vi "TestM1M3SALCommands.vi"() -> ()   [LabVIEW 2016]
uses:
  DataTypes/Topics/Parts/CommandId.ctl
  Communicator/M1M3SAL/M1M3SAL.lvclass
  Communicator/DataTypes/M1M3SALSettings.ctl
  UserEvents/UserEvents.lvclass
  DataTypes/General/ShutdownEvent.ctl
  Communicator/M1M3SAL/M1M3SAL.lvclass/M1M3SAL.ctl
  UserEvents/UserEvents.lvclass/UserEvents.ctl
  Commands/AbortLowerM1M3Command/AbortLowerM1M3Command.lvclass
  Commands/AbortLowerM1M3Command/AbortLowerM1M3Command.lvclass/AbortLowerM1M3Command.ctl
  Commands/AbortRaiseM1M3Command/AbortRaiseM1M3Command.lvclass
  Commands/AbortRaiseM1M3Command/AbortRaiseM1M3Command.lvclass/AbortRaiseM1M3Command.ctl
  Commands/ApplyAberrationByBendingModesCommand/ApplyAberrationByBendingModesCommand.lvclass
  Commands/ApplyAberrationByBendingModesCommand/ApplyAberrationByBendingModesCommand.lvclass/ApplyAberrationByBendingModesCommand.ctl
  Commands/ApplyAberrationByForcesCommand/ApplyAberrationByForcesCommand.lvclass
  Commands/ApplyAberrationByForcesCommand/ApplyAberrationByForcesCommand.lvclass/ApplyAberrationByForcesCommand.ctl
  Commands/ApplyAOSCorrectionByBendingModesCommand/ApplyAOSCorrectionByBendingModesCommand.lvclass
  Commands/ApplyAOSCorrectionByBendingModesCommand/ApplyAOSCorrectionByBendingModesCommand.lvclass/ApplyAOSCorrectionByBendingModesCommand.ctl
  Commands/ApplyAOSCorrectionByForcesCommand/ApplyAOSCorrectionByForcesCommand.lvclass
  Commands/ApplyAOSCorrectionByForcesCommand/ApplyAOSCorrectionByForcesCommand.lvclass/ApplyAOSCorrectionByForcesCommand.ctl
  Commands/ClearAberrationCommand/ClearAberrationCommand.lvclass
  Commands/ClearAberrationCommand/ClearAberrationCommand.lvclass/ClearAberrationCommand.ctl
  Commands/ClearAOSCorrectionCommand/ClearAOSCorrectionCommand.lvclass
  Commands/ClearAOSCorrectionCommand/ClearAOSCorrectionCommand.lvclass/ClearAOSCorrectionCommand.ctl
  Commands/DisableCommand/DisableCommand.lvclass
  Commands/DisableCommand/DisableCommand.lvclass/DisableCommand.ctl
  Commands/EnableCommand/EnableCommand.lvclass
  Commands/EnableCommand/EnableCommand.lvclass/EnableCommand.ctl
  Commands/EnterMaintenanceCommand/EnterMaintenanceCommand.lvclass
  Commands/EnterMaintenanceCommand/EnterMaintenanceCommand.lvclass/EnterMaintenanceCommand.ctl
  Commands/ExitCommand/ExitCommand.lvclass
  Commands/ExitCommand/ExitCommand.lvclass/ExitCommand.ctl
  Commands/ExitMaintenanceCommand/ExitMaintenanceCommand.lvclass
  Commands/ExitMaintenanceCommand/ExitMaintenanceCommand.lvclass/ExitMaintenanceCommand.ctl
  Commands/LowerM1M3Command/LowerM1M3Command.lvclass
  Commands/LowerM1M3Command/LowerM1M3Command.lvclass/LowerM1M3Command.ctl
  Commands/ManipulateM1M3Command/ManipulateM1M3Command.lvclass
  Commands/ManipulateM1M3Command/ManipulateM1M3Command.lvclass/ManipulateM1M3Command.ctl
  Commands/MoveHardpointActuatorsCommand/MoveHardpointActuatorsCommand.lvclass
  Commands/MoveHardpointActuatorsCommand/MoveHardpointActuatorsCommand.lvclass/MoveHardpointActuatorsCommand.ctl
  Commands/RaiseM1M3Command/RaiseM1M3Command.lvclass
  Commands/RaiseM1M3Command/RaiseM1M3Command.lvclass/RaiseM1M3Command.ctl
  Commands/ShutdownCommand/ShutdownCommand.lvclass
  Commands/ShutdownCommand/ShutdownCommand.lvclass/ShutdownCommand.ctl
  Commands/StandbyCommand/StandbyCommand.lvclass
  Commands/StandbyCommand/StandbyCommand.lvclass/StandbyCommand.ctl
  Commands/StartCommand/StartCommand.lvclass
  Commands/StartCommand/StartCommand.lvclass/StartCommand.ctl
  Commands/TestAirCommand/TestAirCommand.lvclass
  Commands/TestAirCommand/TestAirCommand.lvclass/TestAirCommand.ctl
  Commands/TestForceActuatorCommand/TestForceActuatorCommand.lvclass
  Commands/TestForceActuatorCommand/TestForceActuatorCommand.lvclass/TestForceActuatorCommand.ctl
  Commands/TestHardpointCommand/TestHardpointCommand.lvclass
  Commands/TestHardpointCommand/TestHardpointCommand.lvclass/TestHardpointCommand.ctl
  DataTypes/Topics/CommandStart.ctl
  DataTypes/Topics/CommandEnable.ctl
  DataTypes/Topics/CommandDisable.ctl
  DataTypes/Topics/CommandStandby.ctl
  DataTypes/Topics/CommandShutdown.ctl
  DataTypes/Topics/CommandExit.ctl
  DataTypes/Topics/CommandManipulateM1M3.ctl
  DataTypes/Topics/CommandTestAir.ctl
  DataTypes/Topics/CommandEnterMaintenance.ctl
  DataTypes/Topics/CommandExitMaintenance.ctl
  DataTypes/Topics/CommandTestHardpoint.ctl
  DataTypes/Topics/CommandTestForceActuator.ctl
  DataTypes/Topics/CommandMoveHardpointActuators.ctl
  DataTypes/Topics/CommandClearAOSCorrection.ctl
  DataTypes/Topics/CommandApplyAOSCorrectionByBendingModes.ctl
  DataTypes/Topics/CommandApplyAOSCorrectionByForces.ctl
  DataTypes/Topics/CommandAbortLowerM1M3.ctl
  DataTypes/Topics/CommandAbortRaiseM1M3.ctl
  DataTypes/Topics/CommandRaiseM1M3.ctl
  DataTypes/Topics/CommandLowerM1M3.ctl
  DataTypes/Topics/CommandApplyAberrationByForces.ctl
  DataTypes/Topics/CommandApplyAberrationByBendingModes.ctl
  DataTypes/Topics/CommandClearAberration.ctl
  Communicator/M1M3SupportCommunicator.lvlib
  DataTypes/General/M1M3SupportGeneral.lvlib
  DataTypes/Topics/M1M3SupportTopics.lvlib
  Commands/Command/Command.lvclass
panel:
  out "CommandId":T1
  out "SAL Start Time (s)":dbl format="%.6g"
  out "ClearAberration":bool
  out "ApplyAberrationBModes":bool
  out "ApplyAberrationForces":bool
  out "Lower":bool
  out "Raise":bool
  out "AbortRaise":bool
  out "AbortLower":bool
  out "ApplyAOSForces":bool
  out "ApplyAOSBModes":bool
  out "ClearAOSCorrection":bool
  out "MoveHardpointActuators":bool
  out "TestForceActuator":bool
  out "TestHardpoint":bool
  in  "ClearAberrationGo":bool
  in  "ApplyAberrationBModesGo":bool
  in  "ApplyAberrationForcesGo":bool
  in  "LowerGo":bool
  in  "RaiseGo":bool
  in  "AbortRaiseGo":bool
  in  "AbortLowerGo":bool
  in  "ApplyAOSForcesGo":bool
  in  "ApplyAOSBModesGo":bool
  in  "ClearAOSCorrectionGo":bool
  in  "MoveHardpointActuatorsGo":bool
  in  "TestForceActuatorGo":bool
  in  "TestHardpointGo":bool
  out "TestAir":bool
  in  "TestAirGo":bool
  out "ExitMaintenance":bool
  out "EnterMaintenance":bool
  out "ManipulateM1M3":bool
  in  "ExitMaintenanceGo":bool
  in  "EnterMaintenanceGo":bool
  in  "ManipulateM1M3Go":bool
  out "Exit":bool
  out "Shutdown":bool
  out "Standby":bool
  out "Disable":bool
  in  "ExitGo":bool
  in  "ShutdownGo":bool
  in  "StandbyGo":bool
  in  "DisableGo":bool
  in  "EnableGo":bool
  out "Enable":bool
  out "Ready?":bool
  in  "StartGo":bool
  out "Start":bool
  in  "Stop":bool
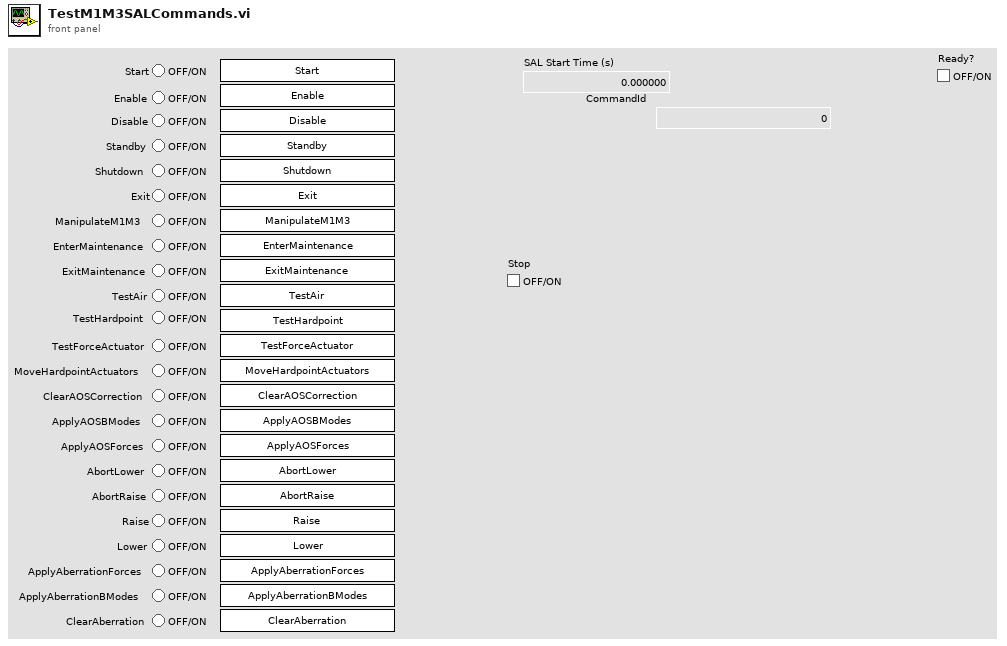
[diagram p1: front panel]
types:
  T1 = typedef "M1M3SupportTopics.lvlib/CommandId.ctl" = i32
  T2 = typedef "M1M3SupportGeneral.lvlib/ShutdownEvent.ctl" = cluster{"Shutdown":bool}
  T3 = typedef "M1M3SupportCommunicator.lvlib/M1M3SALSettings.ctl" = cluster{"IPAddress":string, "Port":u16, "StartupScript":string}
  T4 = typedef "M1M3SupportTopics.lvlib/CommandAbortLowerM1M3.ctl" = cluster{"CommandId":T1, "AbortLowerM1M3":bool}
  T5 = typedef "M1M3SupportTopics.lvlib/CommandAbortRaiseM1M3.ctl" = cluster{"CommandId":T1, "AbortRaiseM1M3":bool}
  T6 = typedef "M1M3SupportTopics.lvlib/CommandApplyAberrationByBendingModes.ctl" = cluster{"CommandId":T1, "Coefficients":dbl[]}
  T7 = typedef "M1M3SupportTopics.lvlib/CommandApplyAberrationByForces.ctl" = cluster{"CommandId":T1, "ZForces":dbl[]}
  T8 = typedef "M1M3SupportTopics.lvlib/CommandApplyAOSCorrectionByBendingModes.ctl" = cluster{"CommandId":T1, "Coefficients":dbl[]}
  T9 = typedef "M1M3SupportTopics.lvlib/CommandApplyAOSCorrectionByForces.ctl" = cluster{"CommandId":T1, "ZForces":dbl[]}
  T10 = typedef "M1M3SupportTopics.lvlib/CommandClearAberration.ctl" = cluster{"CommandId":T1, "ClearAberration":bool}
  T11 = typedef "M1M3SupportTopics.lvlib/CommandClearAOSCorrection.ctl" = cluster{"CommandId":T1, "ClearAOSCorrection":bool}
  T12 = typedef "M1M3SupportTopics.lvlib/CommandDisable.ctl" = cluster{"CommandId":T1, "Disable":bool}
  T13 = typedef "M1M3SupportTopics.lvlib/CommandEnable.ctl" = cluster{"CommandId":T1, "Enable":bool}
  T14 = typedef "M1M3SupportTopics.lvlib/CommandEnterMaintenance.ctl" = cluster{"CommandId":T1, "EnterMaintenance":bool}
  T15 = typedef "M1M3SupportTopics.lvlib/CommandExit.ctl" = cluster{"CommandId":T1, "Exit":bool}
  T16 = typedef "M1M3SupportTopics.lvlib/CommandExitMaintenance.ctl" = cluster{"CommandId":T1, "ExitMaintenance":bool}
  T17 = typedef "M1M3SupportTopics.lvlib/CommandLowerM1M3.ctl" = cluster{"CommandId":T1, "LowerM1M3":bool}
  T18 = typedef "M1M3SupportTopics.lvlib/CommandManipulateM1M3.ctl" = cluster{"CommandId":T1, "XTranslation":dbl, "YTranslation":dbl, "ZTranslation":dbl, "XRotation":dbl, "YRotation":dbl, "ZRotation":dbl}
  T19 = typedef "M1M3SupportTopics.lvlib/CommandMoveHardpointActuators.ctl" = cluster{"CommandId":T1, "Steps":i8[]}
  T20 = typedef "M1M3SupportTopics.lvlib/CommandRaiseM1M3.ctl" = cluster{"CommandId":T1, "RaiseM1M3":bool}
  T21 = typedef "M1M3SupportTopics.lvlib/CommandShutdown.ctl" = cluster{"CommandId":T1, "Shutdown":bool}
  T22 = typedef "M1M3SupportTopics.lvlib/CommandStandby.ctl" = cluster{"CommandId":T1, "Standby":bool}
  T23 = typedef "M1M3SupportTopics.lvlib/CommandStart.ctl" = cluster{"CommandId":T1, "Start":bool, "SettingToApply":string}
  T24 = typedef "M1M3SupportTopics.lvlib/CommandTestAir.ctl" = cluster{"CommandId":T1, "TestAir":bool}
  T25 = typedef "M1M3SupportTopics.lvlib/CommandTestForceActuator.ctl" = cluster{"CommandId":T1, "ActuatorId":i32}
  T26 = typedef "M1M3SupportTopics.lvlib/CommandTestHardpoint.ctl" = cluster{"CommandId":T1, "ActuatorId":i32}
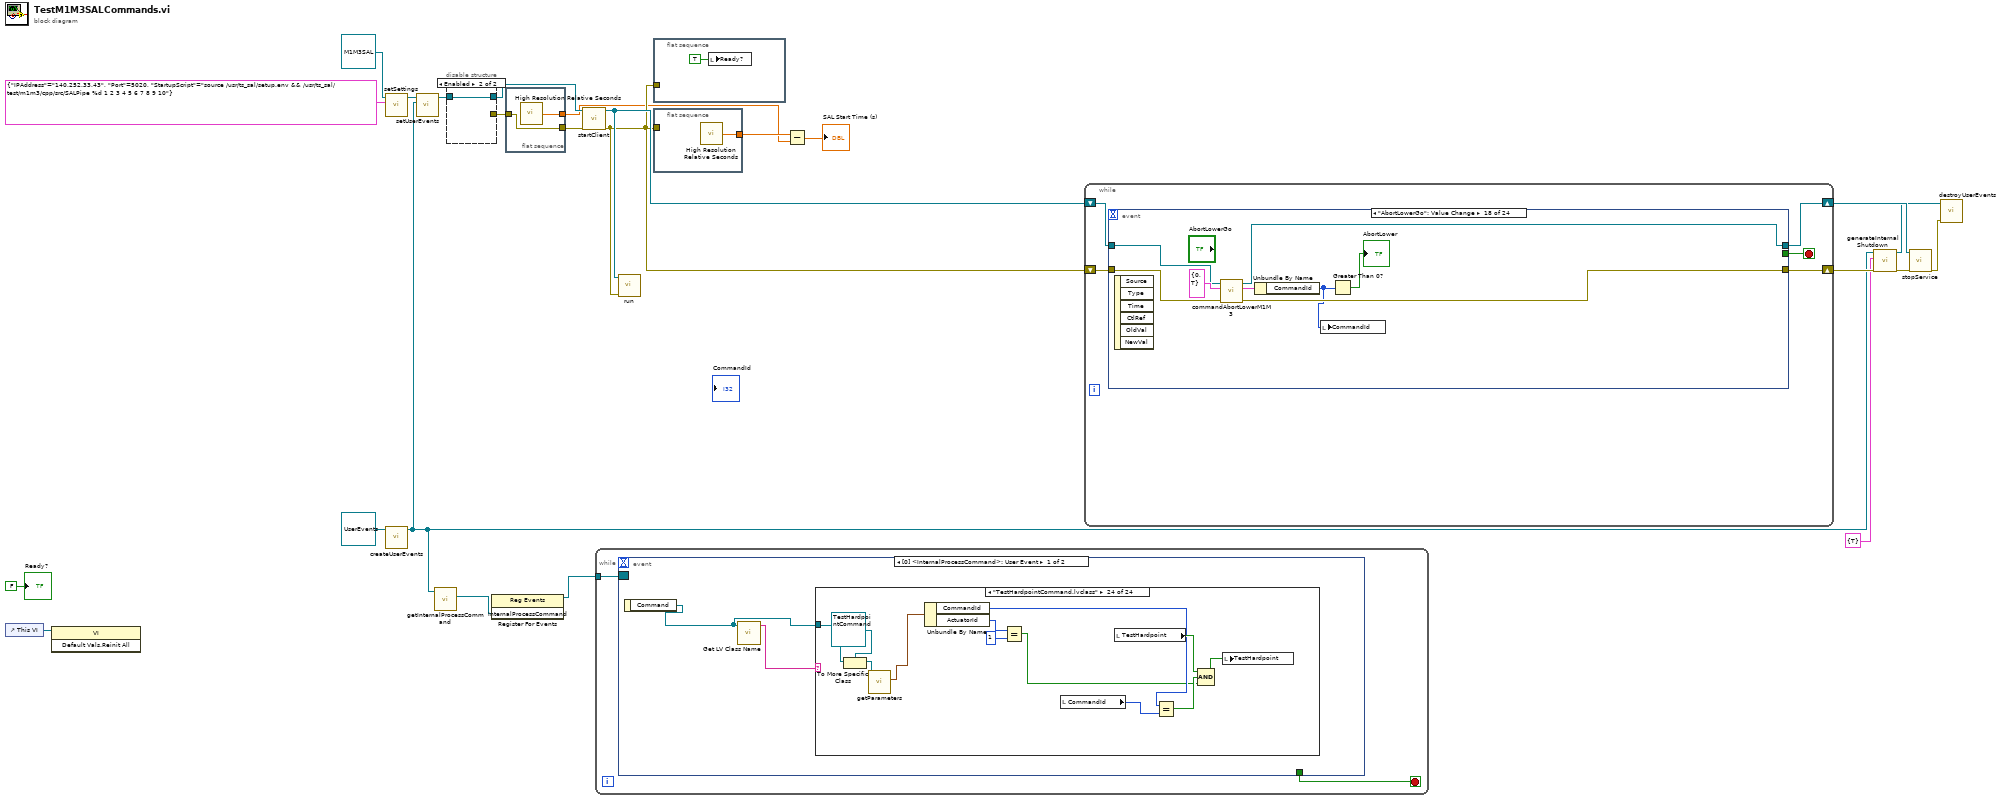
[diagram p0: block diagram]
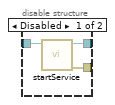
[diagram p2: hidden frame]
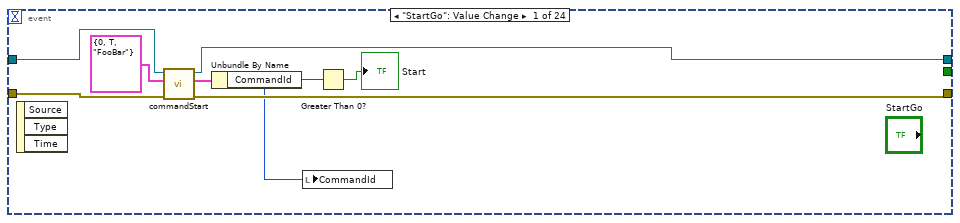
[diagram p3: hidden frame]
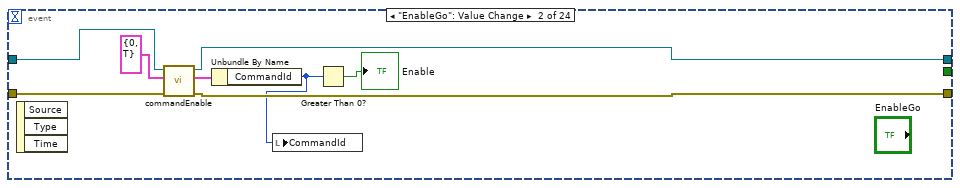
[diagram p4: hidden frame]
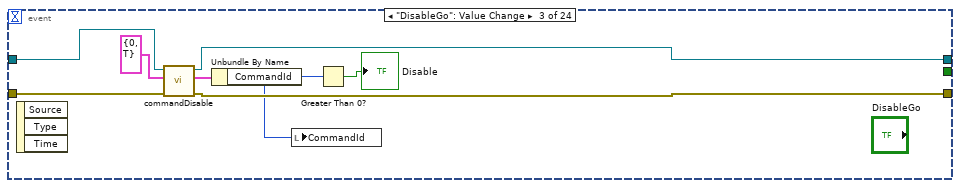
[diagram p5: hidden frame]
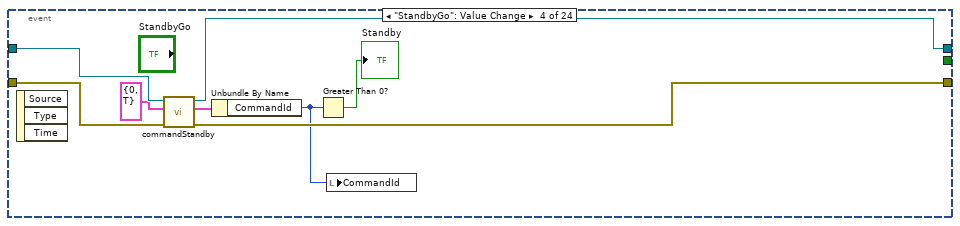
[diagram p6: hidden frame]
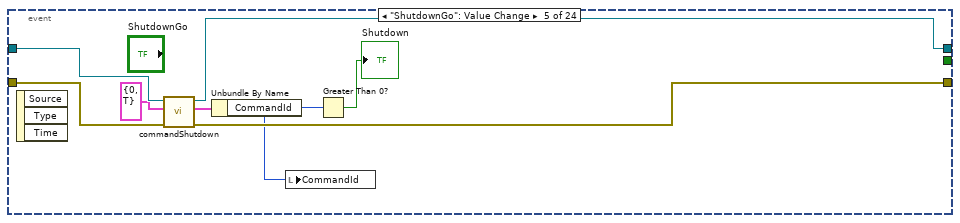
[diagram p7: hidden frame]
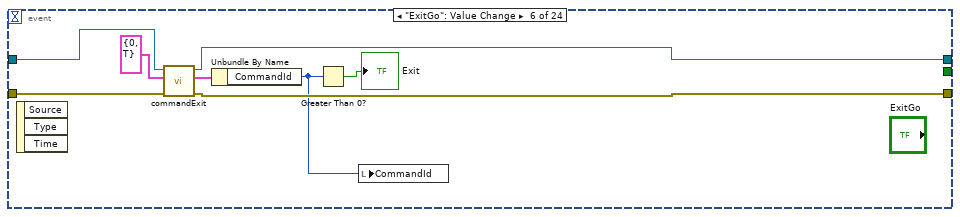
[diagram p8: hidden frame]
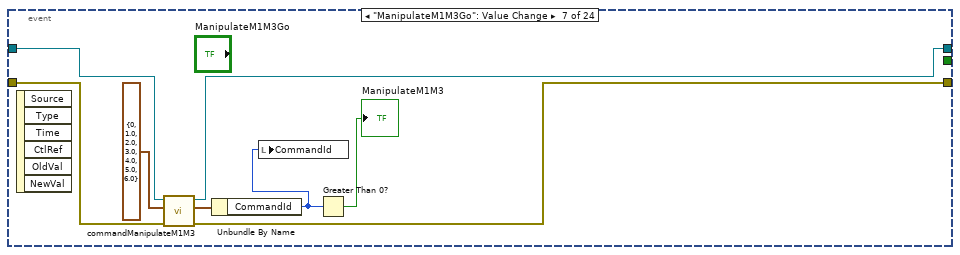
[diagram p9: hidden frame]
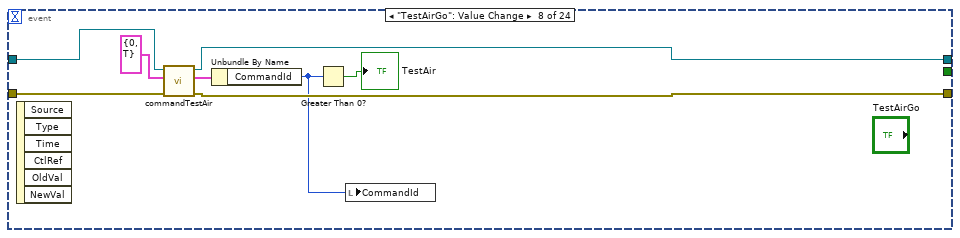
[diagram p10: hidden frame]
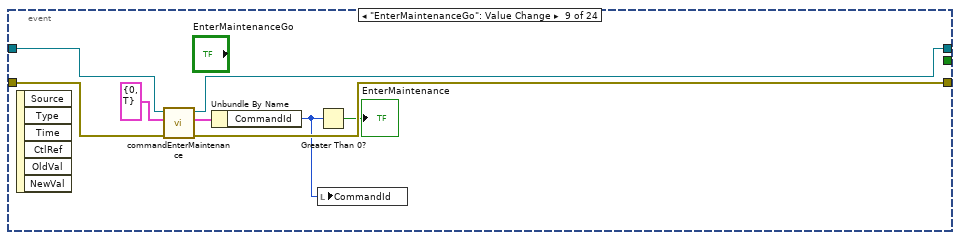
[diagram p11: hidden frame]
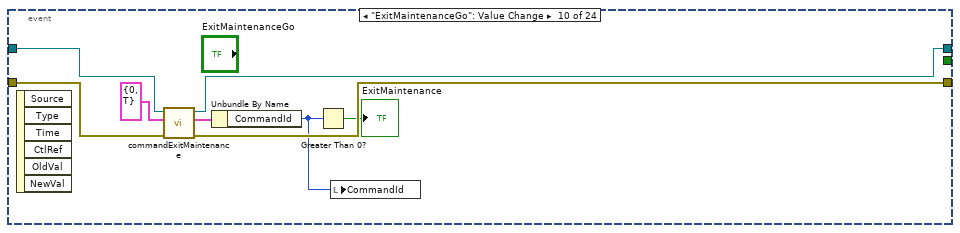
[diagram p12: hidden frame]
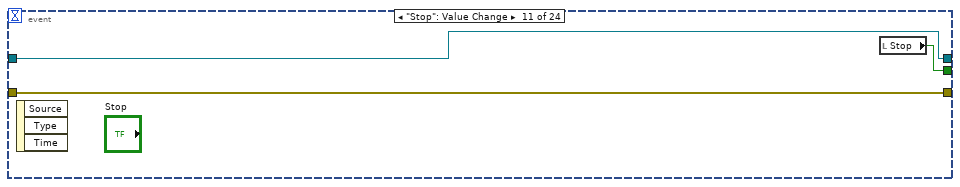
[diagram p13: hidden frame]
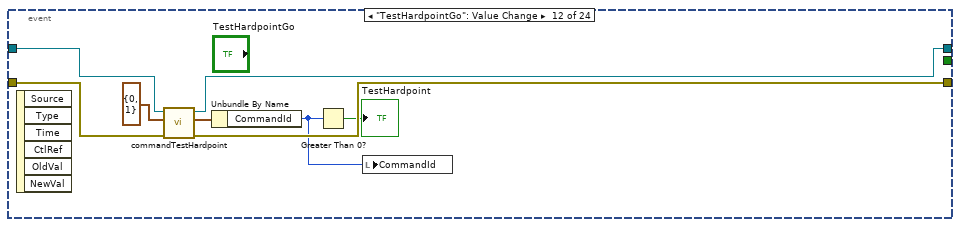
[diagram p14: hidden frame]
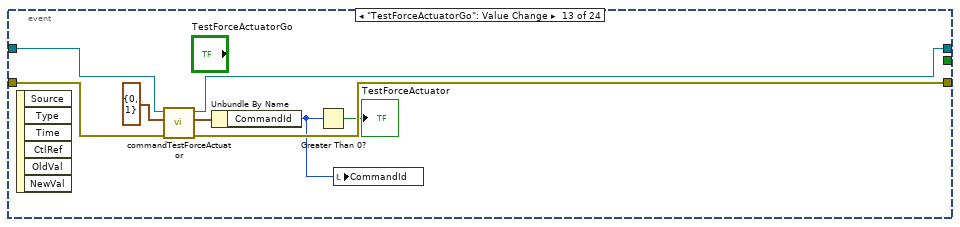
[diagram p15: hidden frame]
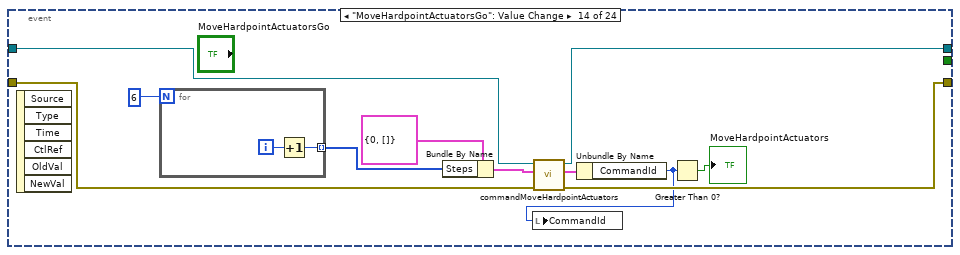
[diagram p16: hidden frame]
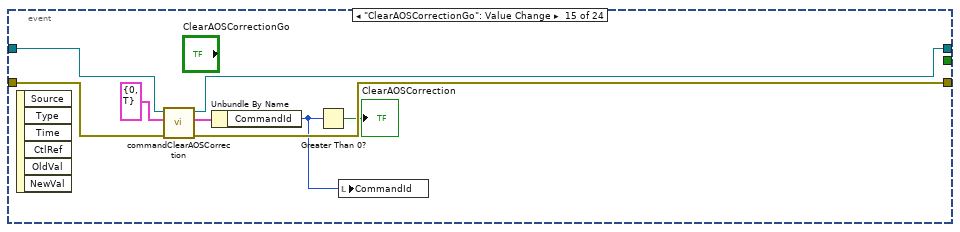
[diagram p17: hidden frame]
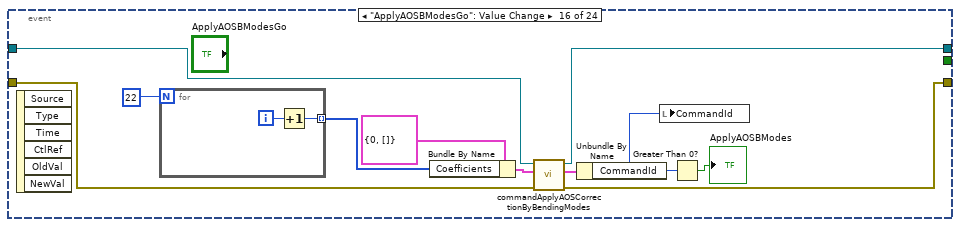
[diagram p18: hidden frame]
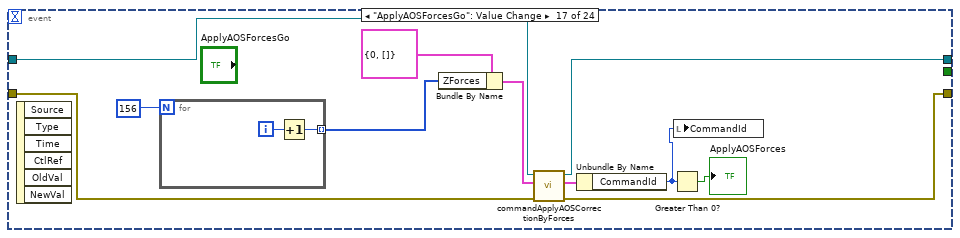
[diagram p19: hidden frame]
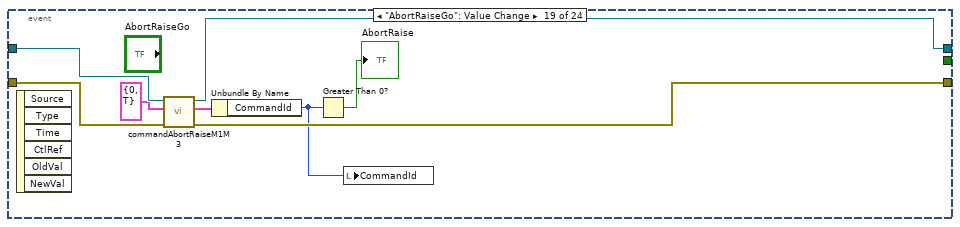
[diagram p20: hidden frame]
diagram:
  n1 = control-ref of="This VI"() -> (w10:refnum<vi>)
  n2 = invoke class="VI" method="Default Vals.Reinit All"(reference=w10) -> ()  [unwired: 2 in, 3 out]
  n3 = call "setSettings.vi"("Settings"=T3 {"IPAddress"="140.252.33.43", "Port"=5020, "StartupScript"="source /usr/ts_sal/setup.env && /usr/ts_sal/test/m1m3/cpp/src/SALPipe %d 1 2 3 4 5 6 7 8 9 10"}, "M1M3SAL in"=refnum<class "M1M3SAL.lvclass"> refnum ("M1M3SupportCommunicator.lvlib:M1M3SAL.lvclass")) -> ("M1M3SAL out"=w21:refnum<class "M1M3SAL.lvclass">)  [unwired: 9 in]
  n4 = call "createUserEvents.vi"("UserEvents in"=refnum<class "UserEvents.lvclass"> refnum ("UserEvents.lvclass")) -> ("UserEvents out"=w3:refnum<class "UserEvents.lvclass">)  [unwired: 9 in, 1 out]
  n5 = call "setUserEvents.vi"("UserEvents"=w3, "M1M3SAL in"=w21) -> ("M1M3SAL out"=w20:refnum<class "M1M3SAL.lvclass">)  [unwired: 9 in]
  n6 = call "getInternalProcessCommand.vi"("UserEvents in"=w3) -> ("InternalProcessCommand"=w2:refnum<user-event>)  [unwired: 9 in, 1 out]
  n7 = disable-structure shown="Enabled" {
    disable-tunnel: w20 -> [w27 w28]
    disable-tunnel: [w26 w28] -> w19
    disable-tunnel: [w25 _] -> w8
    frame Disabled {
      n8 = call-dynamic "startService.vi"("M1M3SAL in"=w27) -> ("error out"=w25:errorcluster, "M1M3SAL out"=w26:refnum<class "M1M3SAL.lvclass">)  [unwired: 9 in]
    }
    frame Enabled {
    }
  }
  n9 = register-events(w2) -> (reference out=w1:refnum<event-registration>)  [unwired: 2 in, 1 out]
  n10 = flat-sequence {
    tunnel: [w30] -> w9
    tunnel: w8 -> [w30]
    tunnel: [w29] -> w5
    frame #0 {
      n11 = call <vilib>:"High Resolution Relative Seconds.vi"() -> ("relative seconds"=w29:dbl)
    }
  }
  n12 = call-dynamic "startClient.vi"("error in (no error)"=w9, "M1M3SAL in"=w19) -> ("error out"=w7:errorcluster, "M1M3SAL out"=w16:refnum<class "M1M3SAL.lvclass">)  [unwired: 8 in]
  n13 = while {
    tunnel: w1 -> [w32]
    stop <- w31 stop-if-true
    n14 = event shown="[0] <InternalProcessCommand>: User Event" {
      selector: w32 -> [_ _]
      dyn-events: _ -> [_ _]
      timeout: _ -> [_ _]
      tunnel: [_ TRUE] -> w31
      event User Event {
        n15 = event-data() -> ("Command"=w33:refnum<class "Command.lvclass">)  [unwired: 1 in]
        n16 = call <vilib>:"Get LV Class Name.vi"("object"=w33) -> ("class name"=w34:string)  [unwired: 9 in, 1 out]
        n17 = case shown="\"TestHardpointCommand.lvclass\"" w34 {
          tunnel: w33 -> [_ w44 w54 w68 w84 w100 w116 w128 w138 w148 w158 w168 w178 w188 w198 w225 w239 w251 w261 w271 w281 w291 w303 w315]
          frame "", Default {
          }
          frame "AbortLowerM1M3Command.lvclass" {
            n18 = To More Specific Class(target class=refnum<class "AbortLowerM1M3Command.lvclass"> refnum ("AbortLowerM1M3Command.lvclass"), reference=w44) -> (specific class reference=w42:refnum<class "AbortLowerM1M3Command.lvclass">)  [unwired: 1 in, 1 out]
            n19 = call "getParameters.vi"("AbortLowerM1M3Command in"=w42) -> ("Parameters"=w41:T4)  [unwired: 9 in, 1 out]
            n20 = local read "CommandId"() -> (w37:T1)
            n21 = Unbundle By Name(w41) -> ("CommandId"=w38:T1, "AbortLowerM1M3"=w40:bool)
            n22 = local read "AbortLower"() -> (w39:bool)
            n23 = Equal?(x=w38, y=w37) -> (x = y?=w36:bool)
            n24 = Compound Arithmetic op=AND(w39, w36, w40) -> (w35:bool)
            n25 = local write "AbortLower"(w35) -> ()
          }
          frame "AbortRaiseM1M3Command.lvclass" {
            n26 = To More Specific Class(target class=refnum<class "AbortRaiseM1M3Command.lvclass"> refnum ("AbortRaiseM1M3Command.lvclass"), reference=w54) -> (specific class reference=w48:refnum<class "AbortRaiseM1M3Command.lvclass">)  [unwired: 1 in, 1 out]
            n27 = call "getParameters.vi"("AbortRaiseM1M3Command in"=w48) -> ("Parameters"=w47:T5)  [unwired: 9 in, 1 out]
            n28 = local read "CommandId"() -> (w52:T1)
            n29 = Unbundle By Name(w47) -> ("CommandId"=w45:T1, "AbortRaiseM1M3"=w46:bool)
            n30 = local read "AbortRaise"() -> (w53:bool)
            n31 = Equal?(x=w45, y=w52) -> (x = y?=w51:bool)
            n32 = Compound Arithmetic op=AND(w53, w51, w46) -> (w50:bool)
            n33 = local write "AbortRaise"(w50) -> ()
          }
          frame "ApplyAberrationByBendingModesCommand.lvclass" {
            n34 = To More Specific Class(target class=refnum<class "ApplyAberrationByBendingModesCommand.lvclass"> refnum ("ApplyAberrationByBendingModesCommand.lvclass"), reference=w68) -> (specific class reference=w61:refnum<class "ApplyAberrationByBendingModesCommand.lvclass">)  [unwired: 1 in, 1 out]
            n35 = for {
              N: 22 -> [_]
              tunnel: [w69] -> w57 mode=indexing
              i -> [w70]
              n36 = Increment(x=w70) -> (x+1=w69:i32)
            }
            n37 = call "getParameters.vi"("ApplyAberrationByBendingModesCommand in"=w61) -> ("Parameters"=w60:T6)  [unwired: 9 in, 1 out]
            n38 = local read "CommandId"() -> (w66:T1)
            n39 = Unbundle By Name(w60) -> ("CommandId"=w63:T1, "Coefficients"=w58:dbl[])
            n40 = Equal?(x=w58, y=w57) -> (x = y?=w56:bool[])
            n41 = And Array Elements(Boolean array=w56) -> (logical AND=w55:bool)
            n42 = local read "ApplyAberrationBModes"() -> (w67:bool)
            n43 = Equal?(x=w63, y=w66) -> (x = y?=w65:bool)
            n44 = Compound Arithmetic op=AND(w67, w65, w55) -> (w64:bool)
            n45 = local write "ApplyAberrationBModes"(w64) -> ()
          }
          frame "ApplyAberrationByForcesCommand.lvclass" {
            n46 = To More Specific Class(target class=refnum<class "ApplyAberrationByForcesCommand.lvclass"> refnum ("ApplyAberrationByForcesCommand.lvclass"), reference=w84) -> (specific class reference=w72:refnum<class "ApplyAberrationByForcesCommand.lvclass">)  [unwired: 1 in, 1 out]
            n47 = call "getParameters.vi"("ApplyAberrationByForcesCommand in"=w72) -> ("Parameters"=w71:T7)  [unwired: 9 in, 1 out]
            n48 = for {
              N: 156 -> [_]
              tunnel: [w85] -> w76 mode=indexing
              i -> [w86]
              n49 = Increment(x=w86) -> (x+1=w85:i32)
            }
            n50 = local read "CommandId"() -> (w82:T1)
            n51 = Unbundle By Name(w71) -> ("CommandId"=w79:T1, "ZForces"=w77:dbl[])
            n52 = Equal?(x=w77, y=w76) -> (x = y?=w75:bool[])
            n53 = And Array Elements(Boolean array=w75) -> (logical AND=w74:bool)
            n54 = local read "ApplyAberrationForces"() -> (w83:bool)
            n55 = Equal?(x=w79, y=w82) -> (x = y?=w81:bool)
            n56 = Compound Arithmetic op=AND(w83, w81, w74) -> (w80:bool)
            n57 = local write "ApplyAberrationForces"(w80) -> ()
          }
          frame "ApplyAOSCorrectionByBendingModesCommand.lvclass" {
            n58 = To More Specific Class(target class=refnum<class "ApplyAOSCorrectionByBendingModesCommand.lvclass"> refnum ("ApplyAOSCorrectionByBendingModesCommand.lvclass"), reference=w100) -> (specific class reference=w88:refnum<class "ApplyAOSCorrectionByBendingModesCommand.lvclass">)  [unwired: 1 in, 1 out]
            n59 = call "getParameters.vi"("ApplyAOSCorrectionByBendingModesCommand in"=w88) -> ("Parameters"=w87:T8)  [unwired: 9 in, 1 out]
            n60 = for {
              N: 22 -> [_]
              tunnel: [w101] -> w92 mode=indexing
              i -> [w102]
              n61 = Increment(x=w102) -> (x+1=w101:i32)
            }
            n62 = local read "CommandId"() -> (w98:T1)
            n63 = Unbundle By Name(w87) -> ("CommandId"=w95:T1, "Coefficients"=w93:dbl[])
            n64 = Equal?(x=w93, y=w92) -> (x = y?=w91:bool[])
            n65 = And Array Elements(Boolean array=w91) -> (logical AND=w90:bool)
            n66 = local read "ApplyAOSBModes"() -> (w99:bool)
            n67 = Equal?(x=w95, y=w98) -> (x = y?=w97:bool)
            n68 = Compound Arithmetic op=AND(w99, w97, w90) -> (w96:bool)
            n69 = local write "ApplyAOSBModes"(w96) -> ()
          }
          frame "ApplyAOSCorrectionByForcesCommand.lvclass" {
            n70 = To More Specific Class(target class=refnum<class "ApplyAOSCorrectionByForcesCommand.lvclass"> refnum ("ApplyAOSCorrectionByForcesCommand.lvclass"), reference=w116) -> (specific class reference=w104:refnum<class "ApplyAOSCorrectionByForcesCommand.lvclass">)  [unwired: 1 in, 1 out]
            n71 = for {
              N: 156 -> [_]
              tunnel: [w117] -> w108 mode=indexing
              i -> [w118]
              n72 = Increment(x=w118) -> (x+1=w117:i32)
            }
            n73 = call "getParameters.vi"("ApplyAOSCorrectionByForcesCommand in"=w104) -> ("Parameters"=w103:T9)  [unwired: 9 in, 1 out]
            n74 = local read "CommandId"() -> (w114:T1)
            n75 = Unbundle By Name(w103) -> ("CommandId"=w111:T1, "ZForces"=w109:dbl[])
            n76 = Equal?(x=w109, y=w108) -> (x = y?=w107:bool[])
            n77 = And Array Elements(Boolean array=w107) -> (logical AND=w106:bool)
            n78 = local read "ApplyAOSForces"() -> (w115:bool)
            n79 = Equal?(x=w111, y=w114) -> (x = y?=w113:bool)
            n80 = Compound Arithmetic op=AND(w115, w113, w106) -> (w112:bool)
            n81 = local write "ApplyAOSForces"(w112) -> ()
          }
          frame "ClearAberrationCommand.lvclass" {
            n82 = To More Specific Class(target class=refnum<class "ClearAberrationCommand.lvclass"> refnum ("ClearAberrationCommand.lvclass"), reference=w128) -> (specific class reference=w121:refnum<class "ClearAberrationCommand.lvclass">)  [unwired: 1 in, 1 out]
            n83 = call "getParameters.vi"("ClearAberrationCommand in"=w121) -> ("Parameters"=w120:T10)  [unwired: 9 in, 1 out]
            n84 = local read "CommandId"() -> (w126:T1)
            n85 = Unbundle By Name(w120) -> ("CommandId"=w123:T1, "ClearAberration"=w119:bool)
            n86 = local read "ClearAberration"() -> (w127:bool)
            n87 = Equal?(x=w123, y=w126) -> (x = y?=w125:bool)
            n88 = Compound Arithmetic op=AND(w127, w125, w119) -> (w124:bool)
            n89 = local write "ClearAberration"(w124) -> ()
          }
          frame "ClearAOSCorrectionCommand.lvclass" {
            n90 = To More Specific Class(target class=refnum<class "ClearAOSCorrectionCommand.lvclass"> refnum ("ClearAOSCorrectionCommand.lvclass"), reference=w138) -> (specific class reference=w129:refnum<class "ClearAOSCorrectionCommand.lvclass">)  [unwired: 1 in, 1 out]
            n91 = call "getParameters.vi"("ClearAOSCorrectionCommand in"=w129) -> ("Parameters"=w131:T11)  [unwired: 9 in, 1 out]
            n92 = local read "CommandId"() -> (w136:T1)
            n93 = Unbundle By Name(w131) -> ("CommandId"=w133:T1, "ClearAOSCorrection"=w132:bool)
            n94 = local read "ClearAOSCorrection"() -> (w137:bool)
            n95 = Equal?(x=w133, y=w136) -> (x = y?=w135:bool)
            n96 = Compound Arithmetic op=AND(w137, w135, w132) -> (w134:bool)
            n97 = local write "ClearAOSCorrection"(w134) -> ()
          }
          frame "DisableCommand.lvclass" {
            n98 = To More Specific Class(target class=refnum<class "DisableCommand.lvclass"> refnum ("DisableCommand.lvclass"), reference=w148) -> (specific class reference=w140:refnum<class "DisableCommand.lvclass">)  [unwired: 1 in, 1 out]
            n99 = call "getParameters.vi"("DisableCommand in"=w140) -> ("Parameters"=w139:T12)  [unwired: 9 in, 1 out]
            n100 = local read "CommandId"() -> (w146:T1)
            n101 = Unbundle By Name(w139) -> ("CommandId"=w143:T1, "Disable"=w142:bool)
            n102 = local read "Disable"() -> (w147:bool)
            n103 = Equal?(x=w143, y=w146) -> (x = y?=w145:bool)
            n104 = Compound Arithmetic op=AND(w147, w145, w142) -> (w144:bool)
            n105 = local write "Disable"(w144) -> ()
          }
          frame "EnableCommand.lvclass" {
            n106 = To More Specific Class(target class=refnum<class "EnableCommand.lvclass"> refnum ("EnableCommand.lvclass"), reference=w158) -> (specific class reference=w150:refnum<class "EnableCommand.lvclass">)  [unwired: 1 in, 1 out]
            n107 = call "getParameters.vi"("EnableCommand in"=w150) -> ("Parameters"=w151:T13)  [unwired: 9 in, 1 out]
            n108 = local read "CommandId"() -> (w156:T1)
            n109 = Unbundle By Name(w151) -> ("CommandId"=w153:T1, "Enable"=w152:bool)
            n110 = local read "Enable"() -> (w157:bool)
            n111 = Equal?(x=w153, y=w156) -> (x = y?=w155:bool)
            n112 = Compound Arithmetic op=AND(w157, w155, w152) -> (w154:bool)
            n113 = local write "Enable"(w154) -> ()
          }
          frame "EnterMaintenanceCommand.lvclass" {
            n114 = To More Specific Class(target class=refnum<class "EnterMaintenanceCommand.lvclass"> refnum ("EnterMaintenanceCommand.lvclass"), reference=w168) -> (specific class reference=w160:refnum<class "EnterMaintenanceCommand.lvclass">)  [unwired: 1 in, 1 out]
            n115 = call "getParameters.vi"("EnterMaintenanceCommand in"=w160) -> ("Parameters"=w159:T14)  [unwired: 9 in, 1 out]
            n116 = local read "CommandId"() -> (w166:T1)
            n117 = Unbundle By Name(w159) -> ("CommandId"=w163:T1, "EnterMaintenance"=w162:bool)
            n118 = local read "EnterMaintenance"() -> (w167:bool)
            n119 = Equal?(x=w163, y=w166) -> (x = y?=w165:bool)
            n120 = Compound Arithmetic op=AND(w167, w165, w162) -> (w164:bool)
            n121 = local write "EnterMaintenance"(w164) -> ()
          }
          frame "ExitCommand.lvclass" {
            n122 = To More Specific Class(target class=refnum<class "ExitCommand.lvclass"> refnum ("ExitCommand.lvclass"), reference=w178) -> (specific class reference=w170:refnum<class "ExitCommand.lvclass">)  [unwired: 1 in, 1 out]
            n123 = call "getParameters.vi"("ExitCommand in"=w170) -> ("Parameters"=w169:T15)  [unwired: 9 in, 1 out]
            n124 = local read "CommandId"() -> (w176:T1)
            n125 = Unbundle By Name(w169) -> ("CommandId"=w173:T1, "Exit"=w172:bool)
            n126 = local read "Exit"() -> (w177:bool)
            n127 = Equal?(x=w173, y=w176) -> (x = y?=w175:bool)
            n128 = Compound Arithmetic op=AND(w177, w175, w172) -> (w174:bool)
            n129 = local write "Exit"(w174) -> ()
          }
          frame "ExitMaintenanceCommand.lvclass" {
            n130 = To More Specific Class(target class=refnum<class "ExitMaintenanceCommand.lvclass"> refnum ("ExitMaintenanceCommand.lvclass"), reference=w188) -> (specific class reference=w180:refnum<class "ExitMaintenanceCommand.lvclass">)  [unwired: 1 in, 1 out]
            n131 = call "getParameters.vi"("ExitMaintenanceCommand in"=w180) -> ("Parameters"=w179:T16)  [unwired: 9 in, 1 out]
            n132 = local read "CommandId"() -> (w186:T1)
            n133 = Unbundle By Name(w179) -> ("CommandId"=w183:T1, "ExitMaintenance"=w182:bool)
            n134 = local read "ExitMaintenance"() -> (w187:bool)
            n135 = Equal?(x=w183, y=w186) -> (x = y?=w185:bool)
            n136 = Compound Arithmetic op=AND(w187, w185, w182) -> (w184:bool)
            n137 = local write "ExitMaintenance"(w184) -> ()
          }
          frame "LowerM1M3Command.lvclass" {
            n138 = To More Specific Class(target class=refnum<class "LowerM1M3Command.lvclass"> refnum ("LowerM1M3Command.lvclass"), reference=w198) -> (specific class reference=w190:refnum<class "LowerM1M3Command.lvclass">)  [unwired: 1 in, 1 out]
            n139 = call "getParameters.vi"("LowerM1M3Command in"=w190) -> ("Parameters"=w189:T17)  [unwired: 9 in, 1 out]
            n140 = local read "CommandId"() -> (w196:T1)
            n141 = Unbundle By Name(w189) -> ("CommandId"=w193:T1, "LowerM1M3"=w192:bool)
            n142 = local read "Lower"() -> (w197:bool)
            n143 = Equal?(x=w193, y=w196) -> (x = y?=w195:bool)
            n144 = Compound Arithmetic op=AND(w197, w195, w192) -> (w194:bool)
            n145 = local write "Lower"(w194) -> ()
          }
          frame "ManipulateM1M3Command.lvclass" {
            n146 = To More Specific Class(target class=refnum<class "ManipulateM1M3Command.lvclass"> refnum ("ManipulateM1M3Command.lvclass"), reference=w225) -> (specific class reference=w218:refnum<class "ManipulateM1M3Command.lvclass">)  [unwired: 1 in, 1 out]
            n147 = call "getParameters.vi"("ManipulateM1M3Command in"=w218) -> ("Parameters"=w217:T18)  [unwired: 9 in, 1 out]
            n148 = Unbundle By Name(w217) -> ("CommandId"=w220:T1, "XTranslation"=w216:dbl, "YTranslation"=w215:dbl, "ZTranslation"=w214:dbl, "XRotation"=w213:dbl, "YRotation"=w212:dbl, "ZRotation"=w211:dbl)
            n149 = Equal?(x=w216, y=1.0) -> (x = y?=w204:bool)
            n150 = Equal?(x=w215, y=2.0) -> (x = y?=w203:bool)
            n151 = Equal?(x=w214, y=3.0) -> (x = y?=w202:bool)
            n152 = Equal?(x=w213, y=4.0) -> (x = y?=w201:bool)
            n153 = Equal?(x=w212, y=5.0) -> (x = y?=w200:bool)
            n154 = Equal?(x=w211, y=6.0) -> (x = y?=w199:bool)
            n155 = local read "CommandId"() -> (w223:T1)
            n156 = local read "ManipulateM1M3"() -> (w224:bool)
            n157 = Equal?(x=w220, y=w223) -> (x = y?=w222:bool)
            n158 = Compound Arithmetic op=AND(w224, w222, w204, w203, w202, w201, w200, w199) -> (w221:bool)
            n159 = local write "ManipulateM1M3"(w221) -> ()
          }
          frame "MoveHardpointActuatorsCommand.lvclass" {
            n160 = To More Specific Class(target class=refnum<class "MoveHardpointActuatorsCommand.lvclass"> refnum ("MoveHardpointActuatorsCommand.lvclass"), reference=w239) -> (specific class reference=w233:refnum<class "MoveHardpointActuatorsCommand.lvclass">)  [unwired: 1 in, 1 out]
            n161 = call "getParameters.vi"("MoveHardpointActuatorsCommand in"=w233) -> ("Parameters"=w232:T19)  [unwired: 9 in, 1 out]
            n162 = Unbundle By Name(w232) -> ("CommandId"=w235:T1, "Steps"=w230:i8[])
            n163 = for {
              N: 6 -> [_]
              tunnel: [w240] -> w229 mode=indexing
              i -> [w241]
              n164 = Increment(x=w241) -> (x+1=w240:i32)
            }
            n165 = Equal?(x=w230, y=w229) -> (x = y?=w228:bool[])
            n166 = And Array Elements(Boolean array=w228) -> (logical AND=w227:bool)
            n167 = local read "CommandId"() -> (w237:T1)
            n168 = local read "MoveHardpointActuators"() -> (w238:bool)
            n169 = Equal?(x=w235, y=w237) -> (x = y?=w236:bool)
            n170 = Compound Arithmetic op=AND(w238, w236, w227) -> (w226:bool)
            n171 = local write "MoveHardpointActuators"(w226) -> ()
          }
          frame "RaiseM1M3Command.lvclass" {
            n172 = To More Specific Class(target class=refnum<class "RaiseM1M3Command.lvclass"> refnum ("RaiseM1M3Command.lvclass"), reference=w251) -> (specific class reference=w244:refnum<class "RaiseM1M3Command.lvclass">)  [unwired: 1 in, 1 out]
            n173 = call "getParameters.vi"("RaiseM1M3Command in"=w244) -> ("Parameters"=w243:T20)  [unwired: 9 in, 1 out]
            n174 = Unbundle By Name(w243) -> ("CommandId"=w247:T1, "RaiseM1M3"=w242:bool)
            n175 = local read "CommandId"() -> (w249:T1)
            n176 = local read "Raise"() -> (w250:bool)
            n177 = Equal?(x=w247, y=w249) -> (x = y?=w248:bool)
            n178 = Compound Arithmetic op=AND(w250, w248, w242) -> (w246:bool)
            n179 = local write "Raise"(w246) -> ()
          }
          frame "ShutdownCommand.lvclass" {
            n180 = To More Specific Class(target class=refnum<class "ShutdownCommand.lvclass"> refnum ("ShutdownCommand.lvclass"), reference=w261) -> (specific class reference=w253:refnum<class "ShutdownCommand.lvclass">)  [unwired: 1 in, 1 out]
            n181 = call "getParameters.vi"("ShutdownCommand in"=w253) -> ("Parameters"=w252:T21)  [unwired: 9 in, 1 out]
            n182 = Unbundle By Name(w252) -> ("CommandId"=w257:T1, "Shutdown"=w255:bool)
            n183 = local read "CommandId"() -> (w259:T1)
            n184 = local read "Shutdown"() -> (w260:bool)
            n185 = Equal?(x=w257, y=w259) -> (x = y?=w258:bool)
            n186 = Compound Arithmetic op=AND(w260, w258, w255) -> (w256:bool)
            n187 = local write "Shutdown"(w256) -> ()
          }
          frame "StandbyCommand.lvclass" {
            n188 = To More Specific Class(target class=refnum<class "StandbyCommand.lvclass"> refnum ("StandbyCommand.lvclass"), reference=w271) -> (specific class reference=w263:refnum<class "StandbyCommand.lvclass">)  [unwired: 1 in, 1 out]
            n189 = call "getParameters.vi"("StandbyCommand in"=w263) -> ("Parameters"=w262:T22)  [unwired: 9 in, 1 out]
            n190 = Unbundle By Name(w262) -> ("CommandId"=w267:T1, "Standby"=w265:bool)
            n191 = local read "CommandId"() -> (w269:T1)
            n192 = local read "Standby"() -> (w270:bool)
            n193 = Equal?(x=w267, y=w269) -> (x = y?=w268:bool)
            n194 = Compound Arithmetic op=AND(w270, w268, w265) -> (w266:bool)
            n195 = local write "Standby"(w266) -> ()
          }
          frame "StartCommand.lvclass" {
            n196 = To More Specific Class(target class=refnum<class "StartCommand.lvclass"> refnum ("StartCommand.lvclass"), reference=w281) -> (specific class reference=w273:refnum<class "StartCommand.lvclass">)  [unwired: 1 in, 1 out]
            n197 = call "getParameters.vi"("StartCommand in"=w273) -> ("Parameters"=w272:T23)  [unwired: 9 in, 1 out]
            n198 = Unbundle By Name(w272) -> ("CommandId"=w277:T1, "Start"=w275:bool)
            n199 = local read "CommandId"() -> (w279:T1)
            n200 = local read "Start"() -> (w280:bool)
            n201 = Equal?(x=w277, y=w279) -> (x = y?=w278:bool)
            n202 = Compound Arithmetic op=AND(w280, w278, w275) -> (w276:bool)
            n203 = local write "Start"(w276) -> ()
          }
          frame "TestAirCommand.lvclass" {
            n204 = To More Specific Class(target class=refnum<class "TestAirCommand.lvclass"> refnum ("TestAirCommand.lvclass"), reference=w291) -> (specific class reference=w283:refnum<class "TestAirCommand.lvclass">)  [unwired: 1 in, 1 out]
            n205 = call "getParameters.vi"("TestAirCommand in"=w283) -> ("Parameters"=w282:T24)  [unwired: 9 in, 1 out]
            n206 = Unbundle By Name(w282) -> ("CommandId"=w287:T1, "TestAir"=w285:bool)
            n207 = local read "CommandId"() -> (w289:T1)
            n208 = local read "TestAir"() -> (w290:bool)
            n209 = Equal?(x=w287, y=w289) -> (x = y?=w288:bool)
            n210 = Compound Arithmetic op=AND(w290, w288, w285) -> (w286:bool)
            n211 = local write "TestAir"(w286) -> ()
          }
          frame "TestForceActuatorCommand.lvclass" {
            n212 = To More Specific Class(target class=refnum<class "TestForceActuatorCommand.lvclass"> refnum ("TestForceActuatorCommand.lvclass"), reference=w303) -> (specific class reference=w296:refnum<class "TestForceActuatorCommand.lvclass">)  [unwired: 1 in, 1 out]
            n213 = call "getParameters.vi"("TestForceActuatorCommand in"=w296) -> ("Parameters"=w295:T25)  [unwired: 9 in, 1 out]
            n214 = Unbundle By Name(w295) -> ("CommandId"=w299:T1, "ActuatorId"=w294:i32)
            n215 = Equal?(x=w294, y=1) -> (x = y?=w292:bool)
            n216 = local read "CommandId"() -> (w301:T1)
            n217 = local read "TestForceActuator"() -> (w302:bool)
            n218 = Equal?(x=w299, y=w301) -> (x = y?=w300:bool)
            n219 = Compound Arithmetic op=AND(w302, w300, w292) -> (w298:bool)
            n220 = local write "TestForceActuator"(w298) -> ()
          }
          frame "TestHardpointCommand.lvclass" {
            n221 = To More Specific Class(target class=refnum<class "TestHardpointCommand.lvclass"> refnum ("TestHardpointCommand.lvclass"), reference=w315) -> (specific class reference=w305:refnum<class "TestHardpointCommand.lvclass">)  [unwired: 1 in, 1 out]
            n222 = call "getParameters.vi"("TestHardpointCommand in"=w305) -> ("Parameters"=w304:T26)  [unwired: 9 in, 1 out]
            n223 = Unbundle By Name(w304) -> ("CommandId"=w311:T1, "ActuatorId"=w309:i32)
            n224 = Equal?(x=w309, y=1) -> (x = y?=w307:bool)
            n225 = local read "CommandId"() -> (w313:T1)
            n226 = local read "TestHardpoint"() -> (w314:bool)
            n227 = Equal?(x=w311, y=w313) -> (x = y?=w312:bool)
            n228 = Compound Arithmetic op=AND(w314, w312, w307) -> (w310:bool)
            n229 = local write "TestHardpoint"(w310) -> ()
          }
        }
      }
      event "Stop": Value Change {
        n230 = event-data() -> ()  [unwired: 1 in, 6 out]
      }
    }
  }
  n231 = call-dynamic "run.vi"("error in (no error)"=w7, "M1M3SAL in"=w16) -> ()  [unwired: 8 in, 2 out]
  n232 = flat-sequence {
    tunnel: w7 -> [_]
    frame #0 {
      n233 = local write "Ready?"(TRUE ("Ready?")) -> ()
    }
  }
  n234 = flat-sequence {
    tunnel: w7 -> [_]
    tunnel: [w318] -> w6
    frame #0 {
      n235 = call <vilib>:"High Resolution Relative Seconds.vi"() -> ("relative seconds"=w318:dbl)
    }
  }
  n236 = Subtract(x=w6, y=w5) -> (x-y=→"SAL Start Time (s)":dbl)
  n237 = while {
    shift-right: [w322] -> w15
    shift-left: w16 -> [w323]
    shift-right: [w320] -> w18
    shift-left: w7 -> [w321]
    stop <- w319 stop-if-true
    n238 = event shown="[17] \"AbortLowerGo\": Value Change" {
      selector: _ -> [_ _ _ _ _ _ _ _ _ _ _ _ _ _ _ _ _ _ _ _ _ _ _ _]
      dyn-events: _ -> [_ _ _ _ _ _ _ _ _ _ _ _ _ _ _ _ _ _ _ _ _ _ _ _]
      timeout: _ -> [_ _ _ _ _ _ _ _ _ _ _ _ _ _ _ _ _ _ _ _ _ _ _ _]
      tunnel: w323 -> [w331 w338 w346 w355 w363 w371 w379 w387 w395 w403 w405 w414 w422 w429 w443 w451 w466 w476 w485 w493 w501 w512 w525 w535]
      tunnel: [w327 w335 w343 w354 w359 w370 w376 w383 w392 w402 w405 w413 w419 w427 w440 w448 w463 w473 w484 w492 w500 w511 w524 w534] -> w322
      tunnel: w321 -> [w329 w337 w345 w352 w362 w368 w378 w385 w394 w400 w404 w411 w421 w428 w442 w450 w465 w475 w482 w491 w499 w510 w522 w533]
      tunnel: [w328 w336 w344 w353 w360 w369 w377 w384 w393 w401 w404 w412 w420 w426 w441 w449 w464 w474 w483 w490 w498 w509 w523 w532] -> w320
      tunnel: [_ _ _ _ _ _ _ _ _ _ w406 _ _ _ _ _ _ _ _ _ _ _ _ _] -> w319
      event "StartGo": Value Change {
        n239 = event-data() -> ()  [unwired: 1 in, 3 out]
        n240 = call-dynamic "commandStart.vi"("error in (no error)"=w329, "CommandStart in"=T23 {"CommandId"=0, "Start"=TRUE, "SettingToApply"="FooBar"}, "M1M3SAL in"=w331) -> ("error out"=w328:errorcluster, "CommandStart out"=w326:T23, "M1M3SAL out"=w327:refnum<class "M1M3SAL.lvclass">)  [unwired: 6 in]
        n241 = Unbundle By Name(w326) -> ("CommandId"=w324:T1)
        n242 = local write "CommandId"(w324) -> ()
        n243 = Greater Than 0?(x=w324) -> (x > 0?=→"Start":bool)
      }
      event "EnableGo": Value Change {
        n244 = event-data() -> ()  [unwired: 1 in, 3 out]
        n245 = call-dynamic "commandEnable.vi"("error in (no error)"=w337, "CommandEnable in"=T13 {"CommandId"=0, "Enable"=TRUE}, "M1M3SAL in"=w338) -> ("error out"=w336:errorcluster, "CommandEnable out"=w334:T13, "M1M3SAL out"=w335:refnum<class "M1M3SAL.lvclass">)  [unwired: 6 in]
        n246 = Unbundle By Name(w334) -> ("CommandId"=w332:T1)
        n247 = local write "CommandId"(w332) -> ()
        n248 = Greater Than 0?(x=w332) -> (x > 0?=→"Enable":bool)
      }
      event "DisableGo": Value Change {
        n249 = event-data() -> ()  [unwired: 1 in, 3 out]
        n250 = call-dynamic "commandDisable.vi"("error in (no error)"=w345, "CommandDisable in"=T12 {"CommandId"=0, "Disable"=TRUE}, "M1M3SAL in"=w346) -> ("error out"=w344:errorcluster, "CommandDisable out"=w342:T12, "M1M3SAL out"=w343:refnum<class "M1M3SAL.lvclass">)  [unwired: 6 in]
        n251 = Unbundle By Name(w342) -> ("CommandId"=w340:T1)
        n252 = local write "CommandId"(w340) -> ()
        n253 = Greater Than 0?(x=w340) -> (x > 0?=→"Disable":bool)
      }
      event "StandbyGo": Value Change {
        n254 = event-data() -> ()  [unwired: 1 in, 3 out]
        n255 = call-dynamic "commandStandby.vi"("error in (no error)"=w352, "CommandStandby in"=T22 {"CommandId"=0, "Standby"=TRUE}, "M1M3SAL in"=w355) -> ("error out"=w353:errorcluster, "CommandStandby out"=w350:T22, "M1M3SAL out"=w354:refnum<class "M1M3SAL.lvclass">)  [unwired: 6 in]
        n256 = Unbundle By Name(w350) -> ("CommandId"=w348:T1)
        n257 = Greater Than 0?(x=w348) -> (x > 0?=→"Standby":bool)
        n258 = local write "CommandId"(w348) -> ()
      }
      event "ShutdownGo": Value Change {
        n259 = event-data() -> ()  [unwired: 1 in, 3 out]
        n260 = call-dynamic "commandShutdown.vi"("error in (no error)"=w362, "CommandShutdown in"=T21 {"CommandId"=0, "Shutdown"=TRUE}, "M1M3SAL in"=w363) -> ("error out"=w360:errorcluster, "CommandShutdown out"=w358:T21, "M1M3SAL out"=w359:refnum<class "M1M3SAL.lvclass">)  [unwired: 6 in]
        n261 = Unbundle By Name(w358) -> ("CommandId"=w356:T1)
        n262 = local write "CommandId"(w356) -> ()
        n263 = Greater Than 0?(x=w356) -> (x > 0?=→"Shutdown":bool)
      }
      event "ExitGo": Value Change {
        n264 = event-data() -> ()  [unwired: 1 in, 3 out]
        n265 = call-dynamic "commandExit.vi"("error in (no error)"=w368, "CommandExit in"=T15 {"CommandId"=0, "Exit"=TRUE}, "M1M3SAL in"=w371) -> ("error out"=w369:errorcluster, "CommandExit out"=w366:T15, "M1M3SAL out"=w370:refnum<class "M1M3SAL.lvclass">)  [unwired: 6 in]
        n266 = Unbundle By Name(w366) -> ("CommandId"=w364:T1)
        n267 = Greater Than 0?(x=w364) -> (x > 0?=→"Exit":bool)
        n268 = local write "CommandId"(w364) -> ()
      }
      event "ManipulateM1M3Go": Value Change {
        n269 = event-data() -> ()  [unwired: 1 in, 6 out]
        n270 = call-dynamic "commandManipulateM1M3.vi"("error in (no error)"=w378, "CommandManipulateM1M3 in"=T18 {"CommandId"=0, "XTranslation"=1.0, "YTranslation"=2.0, "ZTranslation"=3.0, "XRotation"=4.0, "YRotation"=5.0, "ZRotation"=6.0}, "M1M3SAL in"=w379) -> ("error out"=w377:errorcluster, "CommandManipulateM1M3 out"=w374:T18, "M1M3SAL out"=w376:refnum<class "M1M3SAL.lvclass">)  [unwired: 6 in]
        n271 = Unbundle By Name(w374) -> ("CommandId"=w372:T1)
        n272 = local write "CommandId"(w372) -> ()
        n273 = Greater Than 0?(x=w372) -> (x > 0?=→"ManipulateM1M3":bool)
      }
      event "TestAirGo": Value Change {
        n274 = event-data() -> ()  [unwired: 1 in, 6 out]
        n275 = call-dynamic "commandTestAir.vi"("error in (no error)"=w385, "CommandTestAir in"=T24 {"CommandId"=0, "TestAir"=TRUE}, "M1M3SAL in"=w387) -> ("error out"=w384:errorcluster, "CommandTestAir out"=w382:T24, "M1M3SAL out"=w383:refnum<class "M1M3SAL.lvclass">)  [unwired: 6 in]
        n276 = Unbundle By Name(w382) -> ("CommandId"=w380:T1)
        n277 = Greater Than 0?(x=w380) -> (x > 0?=→"TestAir":bool)
        n278 = local write "CommandId"(w380) -> ()
      }
      event "EnterMaintenanceGo": Value Change {
        n279 = event-data() -> ()  [unwired: 1 in, 6 out]
        n280 = call-dynamic "commandEnterMaintenance.vi"("error in (no error)"=w394, "CommandEnterMaintenance in"=T14 {"CommandId"=0, "EnterMaintenance"=TRUE}, "M1M3SAL in"=w395) -> ("error out"=w393:errorcluster, "CommandEnterMaintenance out"=w390:T14, "M1M3SAL out"=w392:refnum<class "M1M3SAL.lvclass">)  [unwired: 6 in]
        n281 = Unbundle By Name(w390) -> ("CommandId"=w388:T1)
        n282 = Greater Than 0?(x=w388) -> (x > 0?=→"EnterMaintenance":bool)
        n283 = local write "CommandId"(w388) -> ()
      }
      event "ExitMaintenanceGo": Value Change {
        n284 = event-data() -> ()  [unwired: 1 in, 6 out]
        n285 = call-dynamic "commandExitMaintenance.vi"("error in (no error)"=w400, "CommandExitMaintenance in"=T16 {"CommandId"=0, "ExitMaintenance"=TRUE}, "M1M3SAL in"=w403) -> ("error out"=w401:errorcluster, "CommandExitMaintenance out"=w398:T16, "M1M3SAL out"=w402:refnum<class "M1M3SAL.lvclass">)  [unwired: 6 in]
        n286 = Unbundle By Name(w398) -> ("CommandId"=w396:T1)
        n287 = Greater Than 0?(x=w396) -> (x > 0?=→"ExitMaintenance":bool)
        n288 = local write "CommandId"(w396) -> ()
      }
      event "Stop": Value Change {
        n289 = event-data() -> ()  [unwired: 1 in, 3 out]
        n290 = local read "Stop"() -> (w406:bool)
      }
      event "TestHardpointGo": Value Change {
        n291 = event-data() -> ()  [unwired: 1 in, 6 out]
        n292 = call-dynamic "commandTestHardpoint.vi"("error in (no error)"=w411, "CommandTestHardpoint in"=T26 {"CommandId"=0, "ActuatorId"=1}, "M1M3SAL in"=w414) -> ("error out"=w412:errorcluster, "CommandTestHardpoint out"=w409:T26, "M1M3SAL out"=w413:refnum<class "M1M3SAL.lvclass">)  [unwired: 6 in]
        n293 = Unbundle By Name(w409) -> ("CommandId"=w407:T1)
        n294 = Greater Than 0?(x=w407) -> (x > 0?=→"TestHardpoint":bool)
        n295 = local write "CommandId"(w407) -> ()
      }
      event "TestForceActuatorGo": Value Change {
        n296 = event-data() -> ()  [unwired: 1 in, 6 out]
        n297 = call-dynamic "commandTestForceActuator.vi"("error in (no error)"=w421, "CommandTestForceActuator in"=T25 {"CommandId"=0, "ActuatorId"=1}, "M1M3SAL in"=w422) -> ("error out"=w420:errorcluster, "CommandTestForceActuator out"=w417:T25, "M1M3SAL out"=w419:refnum<class "M1M3SAL.lvclass">)  [unwired: 6 in]
        n298 = Unbundle By Name(w417) -> ("CommandId"=w415:T1)
        n299 = Greater Than 0?(x=w415) -> (x > 0?=→"TestForceActuator":bool)
        n300 = local write "CommandId"(w415) -> ()
      }
      event "MoveHardpointActuatorsGo": Value Change {
        n301 = event-data() -> ()  [unwired: 1 in, 6 out]
        n302 = for {
          N: 6 -> [_]
          tunnel: [w434] -> w431 mode=indexing
          i -> [w435]
          n303 = Increment(x=w435) -> (x+1=w434:i32)
        }
        n304 = Bundle By Name(cluster=T19 {"CommandId"=0, "Steps"=[]} ("CommandMoveHardpointActuators in"), "Steps"=w431) -> (w430:T19)
        n305 = call-dynamic "commandMoveHardpointActuators.vi"("error in (no error)"=w428, "CommandMoveHardpointActuators in"=w430, "M1M3SAL in"=w429) -> ("error out"=w426:errorcluster, "CommandMoveHardpointActuators out"=w425:T19, "M1M3SAL out"=w427:refnum<class "M1M3SAL.lvclass">)  [unwired: 6 in]
        n306 = Unbundle By Name(w425) -> ("CommandId"=w423:T1)
        n307 = local write "CommandId"(w423) -> ()
        n308 = Greater Than 0?(x=w423) -> (x > 0?=→"MoveHardpointActuators":bool)
      }
      event "ClearAOSCorrectionGo": Value Change {
        n309 = event-data() -> ()  [unwired: 1 in, 6 out]
        n310 = call-dynamic "commandClearAOSCorrection.vi"("error in (no error)"=w442, "CommandClearAOSCorrection in"=T11 {"CommandId"=0, "ClearAOSCorrection"=TRUE}, "M1M3SAL in"=w443) -> ("error out"=w441:errorcluster, "CommandClearAOSCorrection out"=w438:T11, "M1M3SAL out"=w440:refnum<class "M1M3SAL.lvclass">)  [unwired: 6 in]
        n311 = Unbundle By Name(w438) -> ("CommandId"=w436:T1)
        n312 = Greater Than 0?(x=w436) -> (x > 0?=→"ClearAOSCorrection":bool)
        n313 = local write "CommandId"(w436) -> ()
      }
      event "ApplyAOSBModesGo": Value Change {
        n314 = event-data() -> ()  [unwired: 1 in, 6 out]
        n315 = for {
          N: 22 -> [_]
          tunnel: [w455] -> w447 mode=indexing
          i -> [w456]
          n316 = Increment(x=w456) -> (x+1=w455:i32)
        }
        n317 = Bundle By Name(cluster=T8 {"CommandId"=0, "Coefficients"=[]} ("CommandApplyAOSCorrectionByBendingModes in"), "Coefficients"=w447) -> (w452:T8)
        n318 = call-dynamic "commandApplyAOSCorrectionByBendingModes.vi"("error in (no error)"=w450, "CommandApplyAOSCorrectionByBendingModes in"=w452, "M1M3SAL in"=w451) -> ("error out"=w449:errorcluster, "CommandApplyAOSCorrectionByBendingModes out"=w446:T8, "M1M3SAL out"=w448:refnum<class "M1M3SAL.lvclass">)  [unwired: 6 in]
        n319 = Unbundle By Name(w446) -> ("CommandId"=w444:T1)
        n320 = local write "CommandId"(w444) -> ()
        n321 = Greater Than 0?(x=w444) -> (x > 0?=→"ApplyAOSBModes":bool)
      }
      event "ApplyAOSForcesGo": Value Change {
        n322 = event-data() -> ()  [unwired: 1 in, 6 out]
        n323 = for {
          N: 156 -> [_]
          tunnel: [w468] -> w461 mode=indexing
          i -> [w469]
          n324 = Increment(x=w469) -> (x+1=w468:i32)
        }
        n325 = Bundle By Name(cluster=T9 {"CommandId"=0, "ZForces"=[]} ("CommandApplyAOSCorrectionByForces in"), "ZForces"=w461) -> (w460:T9)
        n326 = call-dynamic "commandApplyAOSCorrectionByForces.vi"("error in (no error)"=w465, "CommandApplyAOSCorrectionByForces in"=w460, "M1M3SAL in"=w466) -> ("error out"=w464:errorcluster, "CommandApplyAOSCorrectionByForces out"=w459:T9, "M1M3SAL out"=w463:refnum<class "M1M3SAL.lvclass">)  [unwired: 6 in]
        n327 = Unbundle By Name(w459) -> ("CommandId"=w457:T1)
        n328 = Greater Than 0?(x=w457) -> (x > 0?=→"ApplyAOSForces":bool)
        n329 = local write "CommandId"(w457) -> ()
      }
      event "AbortLowerGo": Value Change {
        n330 = event-data() -> ()  [unwired: 1 in, 6 out]
        n331 = call-dynamic "commandAbortLowerM1M3.vi"("error in (no error)"=w475, "CommandAbortLowerM1M3 in"=T4 {"CommandId"=0, "AbortLowerM1M3"=TRUE}, "M1M3SAL in"=w476) -> ("error out"=w474:errorcluster, "CommandAbortLowerM1M3 out"=w472:T4, "M1M3SAL out"=w473:refnum<class "M1M3SAL.lvclass">)  [unwired: 6 in]
        n332 = Unbundle By Name(w472) -> ("CommandId"=w470:T1)
        n333 = local write "CommandId"(w470) -> ()
        n334 = Greater Than 0?(x=w470) -> (x > 0?=→"AbortLower":bool)
      }
      event "AbortRaiseGo": Value Change {
        n335 = event-data() -> ()  [unwired: 1 in, 6 out]
        n336 = call-dynamic "commandAbortRaiseM1M3.vi"("error in (no error)"=w482, "CommandAbortRaiseM1M3 in"=T5 {"CommandId"=0, "AbortRaiseM1M3"=TRUE}, "M1M3SAL in"=w485) -> ("error out"=w483:errorcluster, "CommandAbortRaiseM1M3 out"=w480:T5, "M1M3SAL out"=w484:refnum<class "M1M3SAL.lvclass">)  [unwired: 6 in]
        n337 = Unbundle By Name(w480) -> ("CommandId"=w478:T1)
        n338 = Greater Than 0?(x=w478) -> (x > 0?=→"AbortRaise":bool)
        n339 = local write "CommandId"(w478) -> ()
      }
      event "RaiseGo": Value Change {
        n340 = event-data() -> ()  [unwired: 1 in, 6 out]
        n341 = call-dynamic "commandRaiseM1M3.vi"("error in (no error)"=w491, "CommandRaiseM1M3 in"=T20 {"CommandId"=0, "RaiseM1M3"=TRUE}, "M1M3SAL in"=w493) -> ("error out"=w490:errorcluster, "CommandRaiseM1M3 out"=w488:T20, "M1M3SAL out"=w492:refnum<class "M1M3SAL.lvclass">)  [unwired: 6 in]
        n342 = Unbundle By Name(w488) -> ("CommandId"=w486:T1)
        n343 = local write "CommandId"(w486) -> ()
        n344 = Greater Than 0?(x=w486) -> (x > 0?=→"Raise":bool)
      }
      event "LowerGo": Value Change {
        n345 = event-data() -> ()  [unwired: 1 in, 6 out]
        n346 = call-dynamic "commandLowerM1M3.vi"("error in (no error)"=w499, "CommandLowerM1M3 in"=T17 {"CommandId"=0, "LowerM1M3"=TRUE}, "M1M3SAL in"=w501) -> ("error out"=w498:errorcluster, "CommandLowerM1M3 out"=w496:T17, "M1M3SAL out"=w500:refnum<class "M1M3SAL.lvclass">)  [unwired: 6 in]
        n347 = Unbundle By Name(w496) -> ("CommandId"=w494:T1)
        n348 = Greater Than 0?(x=w494) -> (x > 0?=→"Lower":bool)
        n349 = local write "CommandId"(w494) -> ()
      }
      event "ApplyAberrationForcesGo": Value Change {
        n350 = event-data() -> ()  [unwired: 1 in, 6 out]
        n351 = for {
          N: 156 -> [_]
          tunnel: [w513] -> w507 mode=indexing
          i -> [w514]
          n352 = Increment(x=w514) -> (x+1=w513:i32)
        }
        n353 = Bundle By Name(cluster=T7 {"CommandId"=0, "ZForces"=[]} ("CommandApplyAberrationByForces in"), "ZForces"=w507) -> (w505:T7)
        n354 = call-dynamic "commandApplyAberrationByForces.vi"("error in (no error)"=w510, "CommandApplyAberrationByForces in"=w505, "M1M3SAL in"=w512) -> ("error out"=w509:errorcluster, "CommandApplyAberrationByForces out"=w504:T7, "M1M3SAL out"=w511:refnum<class "M1M3SAL.lvclass">)  [unwired: 6 in]
        n355 = Unbundle By Name(w504) -> ("CommandId"=w502:T1)
        n356 = local write "CommandId"(w502) -> ()
        n357 = Greater Than 0?(x=w502) -> (x > 0?=→"ApplyAberrationForces":bool)
      }
      event "ApplyAberrationBModesGo": Value Change {
        n358 = event-data() -> ()  [unwired: 1 in, 6 out]
        n359 = for {
          N: 22 -> [_]
          tunnel: [w526] -> w518 mode=indexing
          i -> [w527]
          n360 = Increment(x=w527) -> (x+1=w526:i32)
        }
        n361 = Bundle By Name(cluster=T6 {"CommandId"=0, "Coefficients"=[]} ("CommandApplyAberrationByBendingModes in"), "Coefficients"=w518) -> (w519:T6)
        n362 = call-dynamic "commandApplyAberrationByBendingModes.vi"("error in (no error)"=w522, "CommandApplyAberrationByBendingModes in"=w519, "M1M3SAL in"=w525) -> ("error out"=w523:errorcluster, "CommandApplyAberrationByBendingModes out"=w517:T6, "M1M3SAL out"=w524:refnum<class "M1M3SAL.lvclass">)  [unwired: 6 in]
        n363 = Unbundle By Name(w517) -> ("CommandId"=w515:T1)
        n364 = local write "CommandId"(w515) -> ()
        n365 = Greater Than 0?(x=w515) -> (x > 0?=→"ApplyAberrationBModes":bool)
      }
      event "ClearAberrationGo": Value Change {
        n366 = event-data() -> ()  [unwired: 1 in, 6 out]
        n367 = call-dynamic "commandClearAberration.vi"("error in (no error)"=w533, "CommandClearAberration in"=T10 {"CommandId"=0, "ClearAberration"=TRUE}, "M1M3SAL in"=w535) -> ("error out"=w532:errorcluster, "CommandClearAberration out"=w530:T10, "M1M3SAL out"=w534:refnum<class "M1M3SAL.lvclass">)  [unwired: 6 in]
        n368 = Unbundle By Name(w530) -> ("CommandId"=w528:T1)
        n369 = local write "CommandId"(w528) -> ()
        n370 = Greater Than 0?(x=w528) -> (x > 0?=→"ClearAberration":bool)
      }
    }
  }
  n371 = call "generateInternalShutdown.vi"("error in (no error)"=w18, "ShutdownEvent"=T2 {"Shutdown"=TRUE}, "UserEvents in"=w3) -> ("error out"=w14:errorcluster, "UserEvents out"=w13:refnum<class "UserEvents.lvclass">)  [unwired: 7 in]
  n372 = call-dynamic "stopService.vi"("error in (no error)"=w14, "M1M3SAL in"=w15) -> ("error out"=w12:errorcluster)  [unwired: 8 in, 1 out]
  n373 = call "destroyUserEvents.vi"("error in (no error)"=w12, "UserEvents in"=w13) -> ()  [unwired: 8 in, 2 out]
  "Ready?" <- FALSE ("Ready?")
